vi "Counter_Clear(CLR).vi"(2 "baud rate (9600)":u32=115200 caption="보 전송속도(9600)", 3 "AXIS":u16(ring) items=["X", "Y", "X,Y"], 4 "Port":refnum<visa-resource-name>="COM4" caption="VISA 리소스 이름") -> (0 "Error Out":errorcluster caption="에러 출력", 1 "VISA out":refnum<visa-resource-name>)   [LabVIEW 2010]
uses:
  <vilib>/Instr/_visa.llb/VISA Flush IO Buffer Mask.ctl
  <vilib>/Instr/_visa.llb/VISA Configure Serial Port (Instr).vi
panel:
  out "Commend Count":u32
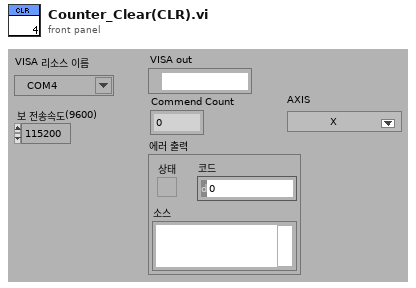
[diagram p1: front panel]
types:
  T1 = typedef "VISA Flush IO Buffer Mask.ctl" = u16
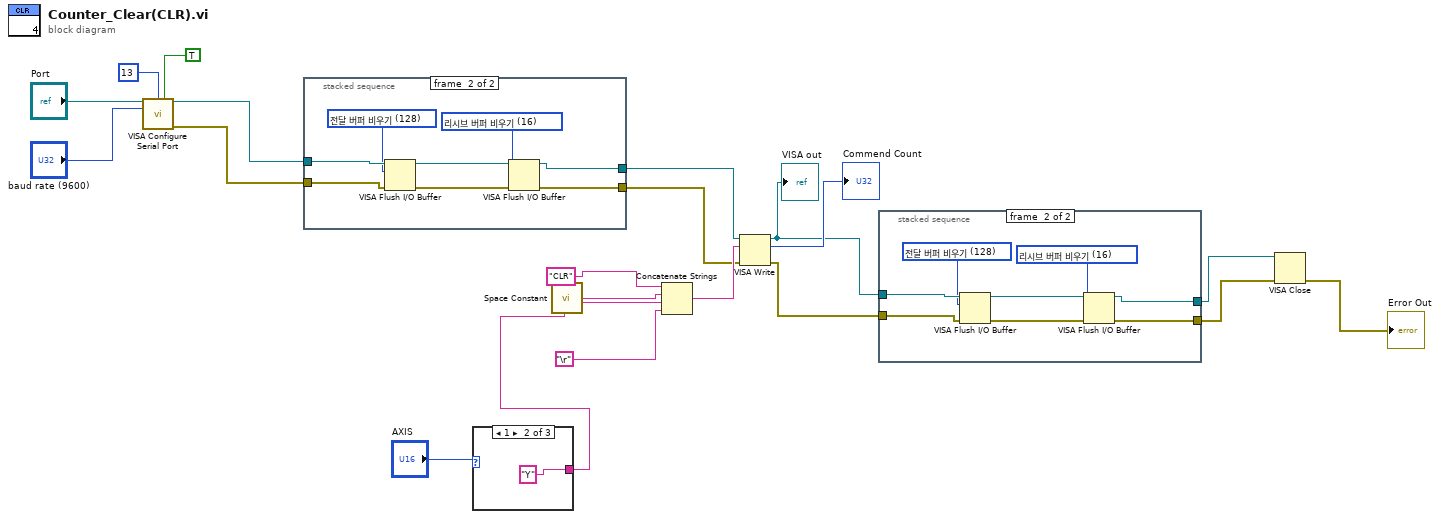
[diagram p0: block diagram]
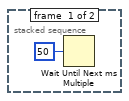
[diagram p2: hidden frame]
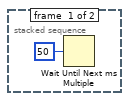
[diagram p3: hidden frame]
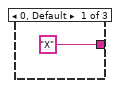
[diagram p4: hidden frame]
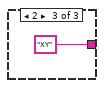
[diagram p5: hidden frame]
diagram:
  n1 = call-poly "VISA Configure Serial Port"("VISA resource name"="Port", "termination char\n(0xA = '\\n' = LF)"=i16 13 ("termination char\n(0xA = '\\n' = LF)"), "Enable Termination\nChar (T)"=TRUE ("Enable Termination\nChar (T)"), "baud rate (9600)"="baud rate (9600)") -> ("VISA resource name out"=w4:refnum<visa-resource-name>, "error out"=w3:errorcluster)  [unwired: 10 in]
  n2 = stacked-sequence {
    tunnel: w4 -> [_ w29]
    tunnel: w3 -> [_ w28]
    tunnel: [_ w24] -> w2
    tunnel: [_ w23] -> w1
    frame #0 {
      n3 = Wait Until Next ms Multiple(millisecond multiple=u32 50 ("ms 배수")) -> ()  [unwired: 1 out]
    }
    frame #1 {
      w22 = T1 16 items=["리시브 버퍼 비우기"=16, "전달 버퍼 디바이스에 쓰기"=32, "리시브 버퍼 비우기(I/O 없음)"=64, "전달 버퍼 비우기"=128] ("Mask")
      w27 = T1 128 items=["리시브 버퍼 비우기"=16, "전달 버퍼 디바이스에 쓰기"=32, "리시브 버퍼 비우기(I/O 없음)"=64, "전달 버퍼 비우기"=128] ("Mask")
      n4 = VISA Flush I/O Buffer(VISA resource name=w29, mask (16)=w27, error in (no error)=w28) -> (VISA resource name out=w26:refnum<visa-resource-name>, error out=w25:errorcluster)
      n5 = VISA Flush I/O Buffer(VISA resource name=w26, mask (16)=w22, error in (no error)=w25) -> (VISA resource name out=w24:refnum<visa-resource-name>, error out=w23:errorcluster)
    }
  }
  n6 = case shown="1" "AXIS" {
    tunnel: ["X" "Y" "XY"] -> w14
    frame 0, Default {
    }
    frame 1 {
    }
    frame 2 {
    }
  }
  n7 = call <vilib>:"Space Constant.vi"() -> ("String"=w19:string)
  n8 = Concatenate Strings("CLR", w19, w14, "\r") -> (w17:string)
  n9 = VISA Write(VISA resource name=w2, write buffer=w17, error in (no error)=w1) -> (VISA resource name out=w8:refnum<visa-resource-name>, return count=→"Commend Count":u32, error out=w7:errorcluster)
  "VISA out" <- w8
  n10 = stacked-sequence {
    tunnel: w8 -> [_ w41]
    tunnel: w7 -> [_ w40]
    tunnel: [_ w36] -> w6
    tunnel: [_ w35] -> w5
    frame #0 {
      n11 = Wait Until Next ms Multiple(millisecond multiple=u32 50 ("ms 배수")) -> ()  [unwired: 1 out]
    }
    frame #1 {
      w34 = T1 16 items=["리시브 버퍼 비우기"=16, "전달 버퍼 디바이스에 쓰기"=32, "리시브 버퍼 비우기(I/O 없음)"=64, "전달 버퍼 비우기"=128] ("Mask")
      w39 = T1 128 items=["리시브 버퍼 비우기"=16, "전달 버퍼 디바이스에 쓰기"=32, "리시브 버퍼 비우기(I/O 없음)"=64, "전달 버퍼 비우기"=128] ("Mask")
      n12 = VISA Flush I/O Buffer(VISA resource name=w41, mask (16)=w39, error in (no error)=w40) -> (VISA resource name out=w38:refnum<visa-resource-name>, error out=w37:errorcluster)
      n13 = VISA Flush I/O Buffer(VISA resource name=w38, mask (16)=w34, error in (no error)=w37) -> (VISA resource name out=w36:refnum<visa-resource-name>, error out=w35:errorcluster)
    }
  }
  n14 = VISA Close(VISA resource name=w6, error in (no error)=w5) -> (error out=→"Error Out":errorcluster)
